vi "NXT_MIDBRAIN Make Dummy Behavior Data.vi"(1 "_sensorData":T1={"_irData"={"_irDistance"=0, "_irHeading"=0, "_irTimestamp"=0}, "_batteryVoltage"=0, "_NXTButtonStates"=[FALSE, FALSE, FALSE]}, 2 "Behavior #":i32, 3 "Behavior Weights":T3=[0, 0, 0, 0, 0, 0]) -> (0 "Behavior Output":T4)   [LabVIEW 2012]
uses:
  SKETCHYDELETINGOFALLTHETHINGS/Tugboat/Robo_Programs/behaviorOutput_t.ctl
  SKETCHYDELETINGOFALLTHETHINGS/Tugboat/Robo_Programs/behaviorWeights_t.ctl
  SKETCHYDELETINGOFALLTHETHINGS/Tugboat/Robo_Programs/sensorData_t.ctl
  SKETCHYDELETINGOFALLTHETHINGS/Tugboat/Robo_Programs/irData_t.ctl
panel:
  # "L\nE\nF\nT"
  # "C\nE\nN\nT\nE\nR"
  # "R\nI\nG\nH\nT"
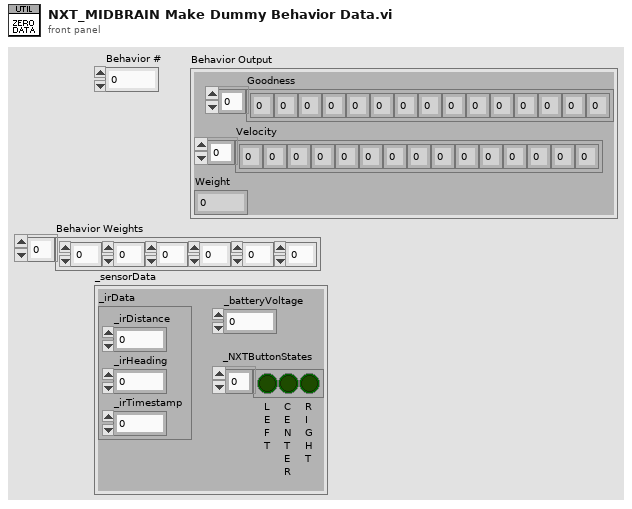
[diagram p1: front panel]
types:
  T1 = typedef "sensorData_t.ctl" = cluster{"_irData":T2, "_batteryVoltage":i32, "_NXTButtonStates":bool[]}
  T2 = typedef "irData_t.ctl" = cluster{"_irDistance":i32, "_irHeading":i32, "_irTimestamp":u32}
  T3 = typedef "behaviorWeights_t.ctl" = i8[]
  T4 = typedef "behaviorOutput_t.ctl" = cluster{"Goodness":i8[], "Velocity":i8[], "Weight":i8}
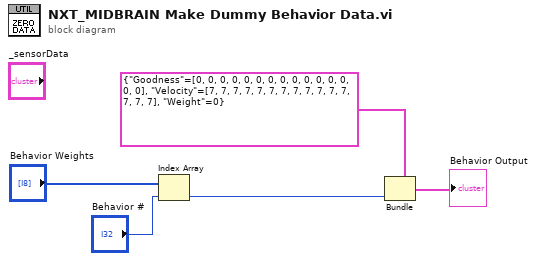
[diagram p0: block diagram]
diagram:
  n1 = Index Array(array="Behavior Weights", index="Behavior #") -> (element=w1:i8)
  n2 = Bundle(cluster=T4 {"Goodness"=[0, 0, 0, 0, 0, 0, 0, 0, 0, 0, 0, 0, 0, 0, 0], "Velocity"=[7, 7, 7, 7, 7, 7, 7, 7, 7, 7, 7, 7, 7, 7, 7], "Weight"=0} ("Behavior Output"), "Weight"=w1) -> (→"Behavior Output":T4)  [unwired: 2 in]
